vi "SVFA Convert FFT Spectrum to Custom Bandwidth Spectrum (1 Ch).vi"(0 "spectrum":cluster{"x0":dbl, "dx":dbl, "magnitude":dbl[]} {"magnitude" format="%.2f"; "dx" format="%.2f"; "x0" format="%.2f"}, 1 "frequency resolution profile in":cluster{"f center":dbl, "bandwidth":dbl}[](array[cluster])=[{"f center"=0.0, "bandwidth"=6.25}, {"f center"=1600.0, "bandwidth"=6.25}, {"f center"=1600.0, "bandwidth"=12.5}, {"f center"=3200.0, "bandwidth"=12.5}, {"f center"=3200.0, "bandwidth"=25.0}, {"f center"=6400.0, "bandwidth"=25.0}, {"f center"=6400.0, "bandwidth"=50.0}, {"f center"=12800.0, "bandwidth"=50.0}, {"f center"=12800.0, "bandwidth"=100.0}, {"f center"=20000.0, "bandwidth"=100.0}], 4 "spectrum info in":T1={"channel name"="", "description"="", "x-axis units"=0, "spectral info"={"spectrum type"=enum."Power [Magnitude^2]", "linear/dB"=enum."linear", "window"=0, "window size"=0, "FFT size"=0}, "engineering units"=0, "custom label"="", "dB reference [EU]"=0.0, "peak units"=enum."rms", "weighting filter"=0, "spectral density?"=FALSE, "unit label"="", "spectrum skewed?"=FALSE, "complimentary spectrum units"=enum."none"} {"x-axis units" items=["Time (s)"=0, "Frequency-CB (Hz)"=1, "Frequency-CPB (Hz)"=1248, "Frequency-Arbitrary (Hz)"=2357, "Quefrency (s)"=2, "Revolutions (rev)"=3, "Order"=4, "Speed (RPM)"=11, "Speed (rad/s)"=21, "Index"=65535]; "weighting filter" items=["Linear", "A-weighting", "B-weighting", "C-weighting", "ITU-R 468-4", "Dolby", "CCITT", "C-message", "Wb", "Wc", "Wd", "We", "Wf", "Wh", "Wj", "Wk", "Wm", "AES17 20 kHz lowpass", "AES17 40 kHz lowpass", "AES17 20 kHz highpass", "AES17 40 kHz highpass"]; "dB reference [EU]" format="%.2f"; "engineering units" items=["custom..."=0, "V"=1, "A"=21, "C"=30, "pC"=31, "s"=32, "-"=29, "Pa"=2, "N"=20, "g"=3, "m/s^2"=4, "m/s"=5, "m"=6, "mm/s"=12, "mm"=13, "micron/s"=14, "micron"=15, "in/s^2"=7, "in/s"=8, "in"=9, "mil/s"=10, "mil"=11, "rad/s^2"=16, "rad/s"=17, "rad"=18, "deg/s^2"=26, "deg/s"=27, "deg"=28, "RPM"=22, "cycle/s^2"=23, "Hz"=24, "cycle"=25, "strain"=19]; "spectral info"."window" items=["None "=0, "Hanning"=1, "Hamming"=2, "Blackman-Harris"=3, "Exact Blackman"=4, "Blackman"=5, "Flat Top"=6, "4 Term B-Harris "=7, "7 Term B-Harris"=8, "Low Sidelobe"=9, "Force - Exponential"=10, "Gaussian"=62]}, 5 "error in (no error)":errorcluster) -> (14 "spectrum":cluster{"frequencies [Hz]":dbl[], "power":dbl[]} {"power" format="%.2f"; "frequencies [Hz]" format="%.2f"}, 15 "unit label":string, 16 "total band power":dbl=nan format="%.2f", 18 "spectrum info out":T1={"channel name"="", "description"="", "x-axis units"=0, "spectral info"={"spectrum type"=enum."Power [Magnitude^2]", "linear/dB"=enum."linear", "window"=0, "window size"=0, "FFT size"=0}, "engineering units"=0, "custom label"="", "dB reference [EU]"=0.0, "peak units"=enum."rms", "weighting filter"=0, "spectral density?"=FALSE, "unit label"="", "spectrum skewed?"=FALSE, "complimentary spectrum units"=enum."none"} {"x-axis units" items=["Time (s)"=0, "Frequency-CB (Hz)"=1, "Frequency-CPB (Hz)"=1248, "Frequency-Arbitrary (Hz)"=2357, "Quefrency (s)"=2, "Revolutions (rev)"=3, "Order"=4, "Speed (RPM)"=11, "Speed (rad/s)"=21, "Index"=65535]; "weighting filter" items=["Linear", "A-weighting", "B-weighting", "C-weighting", "ITU-R 468-4", "Dolby", "CCITT", "C-message", "Wb", "Wc", "Wd", "We", "Wf", "Wh", "Wj", "Wk", "Wm", "AES17 20 kHz lowpass", "AES17 40 kHz lowpass", "AES17 20 kHz highpass", "AES17 40 kHz highpass"]; "dB reference [EU]" format="%.2f"; "engineering units" items=["custom..."=0, "V"=1, "A"=21, "C"=30, "pC"=31, "s"=32, "-"=29, "Pa"=2, "N"=20, "g"=3, "m/s^2"=4, "m/s"=5, "m"=6, "mm/s"=12, "mm"=13, "micron/s"=14, "micron"=15, "in/s^2"=7, "in/s"=8, "in"=9, "mil/s"=10, "mil"=11, "rad/s^2"=16, "rad/s"=17, "rad"=18, "deg/s^2"=26, "deg/s"=27, "deg"=28, "RPM"=22, "cycle/s^2"=23, "Hz"=24, "cycle"=25, "strain"=19]; "spectral info"."window" items=["None "=0, "Hanning"=1, "Hamming"=2, "Blackman-Harris"=3, "Exact Blackman"=4, "Blackman"=5, "Flat Top"=6, "4 Term B-Harris "=7, "7 Term B-Harris"=8, "Low Sidelobe"=9, "Force - Exponential"=10, "Gaussian"=62]}, 19 "error out":errorcluster)   [LabVIEW 2017]
doc: "Computes the aggregate power in the <B>range</B>. The SVL Power in Band VI operates on Power, PSD, COP, and FFT [Mag] spectra. You can use this polymorphic VI to analyze a single spectrum or N spectra. The data type you wire to the <B>spectrum</B> input determines the polymorphic instance to use."
uses:
  <vilib>/addons/_NISVFA/_Shared subVIs/Controls/svc_Spectrum Info.ctl
  <vilib>/addons/_NISVFA/_Shared subVIs/Controls/svc_X-Axis Units.ctl
  <vilib>/addons/_NISVFA/_Shared subVIs/Controls/svc_Spectrum Type.ctl
  <vilib>/addons/_NISVFA/_Shared subVIs/Controls/svc_Engineering Units Text Ring.ctl
  <vilib>/addons/_NISVFA/_Shared subVIs/Controls/svc_Weighting Filter Text Ring.ctl
  <vilib>/addons/_NISVFA/_Shared subVIs/Controls/svc_Complimentary Spectrum Units.ctl
  <vilib>/addons/_NISVFA/_Spectrum Processing/SVFA Unit Conversion (1 Ch).vi
  <vilib>/addons/_NISVFA/_Spectrum Processing/subVIs/svfa_Conversion Utility (spectrum info).vi
  <vilib>/addons/_NISVFA/_Spectrum Processing/subVIs/svfa_Peak to RMS to Peak2Peak.vi
  <vilib>/addons/_NISVFA/_Spectrum Processing/subVIs/svfa_Mag to Mag2.vi
  <vilib>/addons/_NISVFA/_Spectrum Processing/subVIs/svfa_Linear to dB.vi
  <vilib>/addons/_NISVFA/_Spectrum Processing/subVIs/svfa_dBrefA to dBrefB.vi
  <vilib>/addons/_NISVFA/_Spectrum Processing/subVIs/svfa_Spectrum to Spectral Density.vi
  <vilib>/addons/_NISVFA/_Shared subVIs/Common/svc_Get Weighting Enum and Labels.vi
  <vilib>/addons/_NISVFA/_Shared subVIs/Common/svc_Unit Label Lexical Class.vi
  <vilib>/addons/_NISVFA/_Shared subVIs/Common/svc_Engineering Units to Unit Label.vi
  <vilib>/addons/_NISVFA/_Shared subVIs/Common/svc_Format Value (DBL).vi
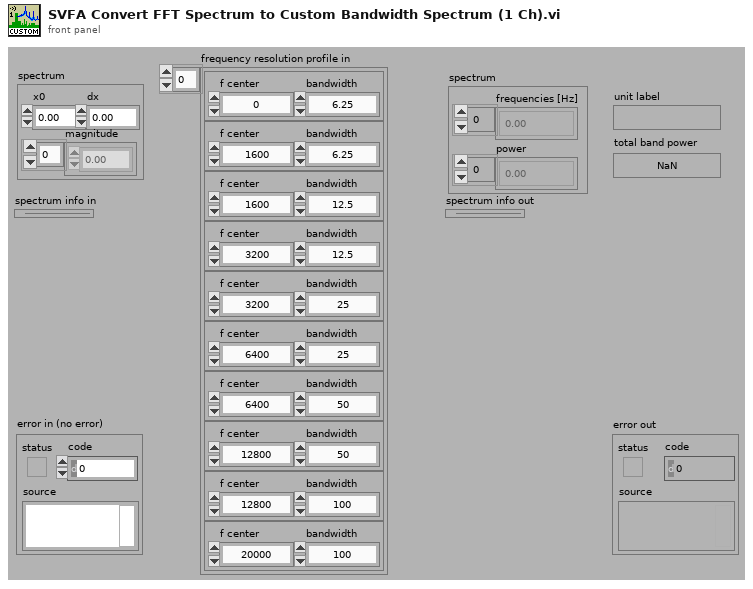
[diagram p1: front panel]
types:
  T1 = typedef "svc_Spectrum Info.ctl" = cluster{"channel name":string, "description":string, "x-axis units":T2, "spectral info":cluster{"spectrum type":T3, "linear/dB":enum16{"linear", "dB"}, "window":u16, "window size":i32, "FFT size":i32}, "engineering units":T4, "custom label":string, "dB reference [EU]":dbl, "peak units":enum16{"rms", "peak", "peak-peak"}, "weighting filter":T5, "spectral density?":bool, "unit label":string, "spectrum skewed?":bool, "complimentary spectrum units":T6}
  T2 = typedef "svc_X-Axis Units.ctl" = u16
  T3 = typedef "svc_Spectrum Type.ctl" = enum16{"FFT Spectrum [complex]", "Amplitude [Magnitude]", "Power [Magnitude^2]", "Cross Spectrum [complex]", "Frequency Response [Complex]"}
  T4 = typedef "svc_Engineering Units Text Ring.ctl" = u16
  T5 = typedef "svc_Weighting Filter Text Ring.ctl" = u16
  T6 = typedef "svc_Complimentary Spectrum Units.ctl" = enum16{"none", "radians", "degrees", "cycles", "imaginary"}
  T7 = cluster{"linear/dB":enum16{"no change", "linear", "dB"}, "dB reference (0: no change)":dbl, "power/magnitude":enum16{"no change", "power", "magnitude"}, "view":enum16{"no change", "rms", "peak", "peak-peak"}}
  T8 = enum16{"no change", "spectrum", "spectral density"}
  T9 = cluster{"f low":dbl, "f high":dbl, "f center":dbl, "bandwidth":dbl}[]
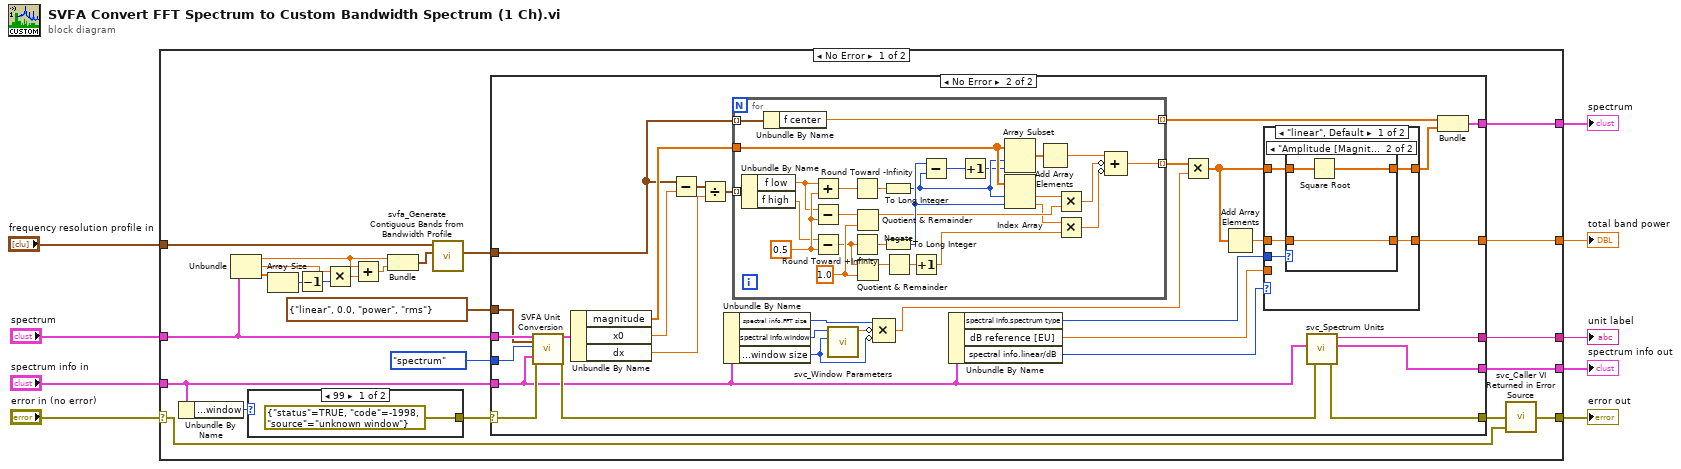
[diagram p0: block diagram]
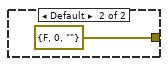
[diagram p2: hidden frame]
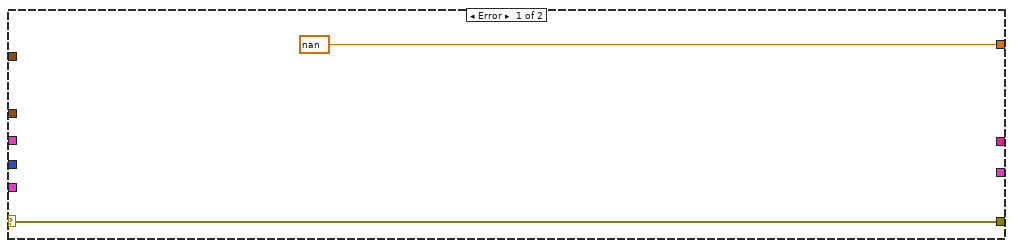
[diagram p3: hidden frame]
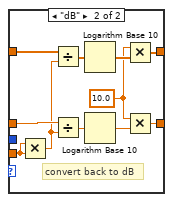
[diagram p5: hidden frame]
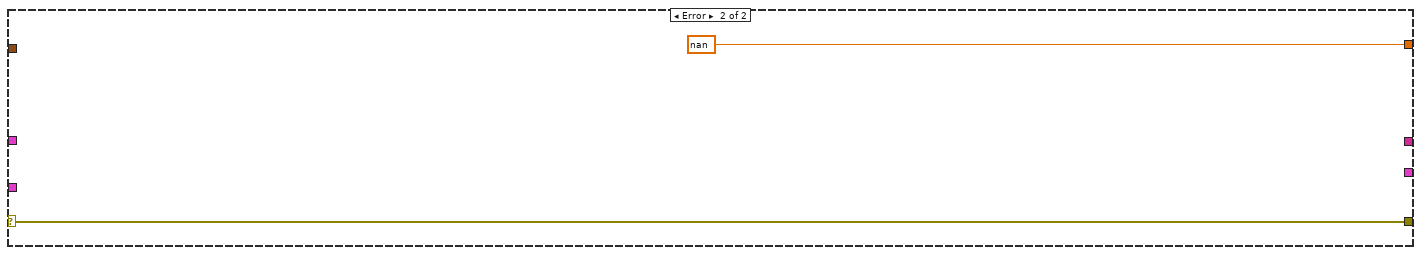
[diagram p6: hidden frame]
diagram:
  n1 = case shown="No Error" "error in (no error)" {
    selector: "error in (no error)" -> [w24 w118]
    tunnel: "spectrum" -> [w20 _]
    tunnel: [w31 nan ("power in band")] -> w8
    tunnel: [w32 w118] -> w7
    tunnel: "spectrum info in" -> [w21 _]
    tunnel: [w18 _] -> w5
    tunnel: [w19 _] -> w3
    tunnel: [w17 _] -> w2
    tunnel: "frequency resolution profile in" -> [w14 _]
    frame No Error {
      n2 = Unbundle By Name(w21) -> ("spectral info.window"=w22:u16)
      n3 = Unbundle(w20) -> ("x0"=w13:dbl, "dx"=w25:dbl, "magnitude"=w29:dbl[])
      n4 = case shown="99" w22 {
        tunnel: [errorcluster {"status"=TRUE, "code"=-1998, "source"="unknown window"} ("error out") errorcluster {"status"=FALSE, "code"=0, "source"=""} ("error out")] -> w23
        frame 99 {
        }
        frame Default {
        }
      }
      n5 = Array Size(array=w29) -> (size(s)=w27:i32)
      n6 = Decrement(x=w27) -> (x-1=w26:i32)
      n7 = Multiply(x=w25, y=w26) -> (x*y=w28:dbl)
      n8 = Add(x=w13, y=w28) -> (x+y=w12:dbl)
      n9 = Bundle("x0"=w13, w12) -> (w11:cluster{"x0":dbl, dbl})  [unwired: 1 in]
      n10 = call <vilib>:"svfa_Generate Contiguous Bands from Bandwidth Profile.vi"("frequency range [Hz]"=w11, "frequency resolution profile in"=w14) -> ("band specifications [Hz]"=w10:T9)  [unwired: 8 in, 1 out]
      n11 = case shown="No Error" w23 {
        selector: w23 -> [w36 w59]
        tunnel: w20 -> [_ w65]
        tunnel: w21 -> [_ w37]
        tunnel: [nan w60] -> w31
        tunnel: [w36 w40] -> w30
        tunnel: [_ w58] -> w19
        tunnel: [_ w41] -> w18
        tunnel: [_ w42] -> w17
        tunnel: T7 {"linear/dB"=enum."linear", "dB reference (0: no change)"=0.0, "power/magnitude"=enum."power", "view"=enum."rms"} ("desired scaling") -> [_ w57]
        tunnel: T8."spectrum" ("spectral density desired") -> [_ w56]
        tunnel: w10 -> [_ w39]
        frame Error {
        }
        frame No Error {
          n12 = call-poly <vilib>:"SVFA Unit Conversion.vi"("spectrum"=w65, "desired scaling"=w57, "spectral density desired"=w56, "spectrum info in"=w37, "error in (no error)"=w59) -> ("converted spectrum"=w67:cluster{"x0":dbl, "dx":dbl, "magnitude":dbl[]}, "error out"=w43:errorcluster)  [unwired: 11 in, 2 out]
          n13 = Unbundle By Name(w67) -> ("magnitude"=w46:dbl[], "x0"=w64:dbl, "dx"=w63:dbl)
          n14 = Subtract(x=w39, y=w64) -> (x-y=w66:T9)
          n15 = Divide(x=w66, y=w63) -> (x/y=w47:T9)
          n16 = Unbundle By Name(w37) -> ("spectral info.FFT size"=w52:i32, "spectral info.window"=w53:u16, "spectral info.window size"=w50:i32)
          n17 = for {
            tunnel: w47 -> [w95] mode=indexing
            tunnel: w46 -> [w94]
            tunnel: [w93] -> w45 mode=indexing
            tunnel: w39 -> [w76] mode=indexing
            tunnel: [w75] -> w38 mode=indexing
            w84 = 0.5 ("x")
            w88 = 1.0 ("y")
            n18 = Unbundle By Name(w95) -> ("f low"=w77:dbl, "f high"=w78:dbl)
            n19 = Unbundle By Name(w76) -> ("f center"=w75:dbl)
            n20 = Add(x=w77, y=w84) -> (x+y=w91:dbl)
            n21 = Subtract(x=w77, y=w84) -> (x-y=w85:dbl)
            n22 = Subtract(x=w78, y=w84) -> (x-y=w81:dbl)
            n23 = Round Toward -Infinity(1:w91) -> (0:w90:dbl)
            n24 = Round Toward +Infinity(x=w81) -> (ceil(x): smallest int >= x=w92:dbl)
            n25 = Quotient & Remainder(x=w85, y=w88) -> (x-y*floor(x/y)=w80:dbl)  [unwired: 1 out]
            n26 = Quotient & Remainder(x=w81, y=w88) -> (x-y*floor(x/y)=w83:dbl)  [unwired: 1 out]
            n27 = To Long Integer(number=w90) -> (32bit integer=w87:i32)
            n28 = To Long Integer(number=w92) -> (32bit integer=w89:i32)
            n29 = Negate(x=w83) -> (-x=w82:dbl)
            n30 = Increment(x=w82) -> (x+1=w79:dbl)
            n31 = Subtract(x=w89, y=w87) -> (x-y=w86:i32)
            n32 = Increment(x=w86) -> (x+1=w70:i32)
            n33 = Array Subset(array=w94, index=w87, length=w70) -> (w71:dbl[])
            n34 = Index Array(array=w94, index #1=w87, index #2=w89) -> (element #1=w69:dbl, element #2=w68:dbl)
            n35 = Add Array Elements(numeric array=w71) -> (sum=w74:dbl)
            n36 = Multiply(x=w69, y=w80) -> (x*y=w73:dbl)
            n37 = Multiply(x=w68, y=w79) -> (x*y=w72:dbl)
            n38 = Compound Arithmetic op=ADD(w74, invert w73, invert w72) -> (w93:dbl)
          }
          n39 = call <vilib>:"svc_Window Parameters.vi"("window size"=w50, "window"=w53) -> ("ENBW"=w51:dbl)  [unwired: 6 in, 3 out]
          n40 = Compound Arithmetic op=MULTIPLY(w52, invert w51, invert w50) -> (w49:dbl)
          n41 = Unbundle By Name(w37) -> ("spectral info.spectrum type"=w44:T3, "dB reference [EU]"=w55:dbl, "spectral info.linear/dB"=w54:enum16{"linear", "dB"})
          n42 = Multiply(x=w45, y=w49) -> (x*y=w48:dbl[])
          n43 = Add Array Elements(numeric array=w48) -> (sum=w61:dbl)
          n44 = case shown="\"linear\", Default" w54 {
            tunnel: [w97 w116] -> w62
            tunnel: w48 -> [w98 w114]
            tunnel: w55 -> [_ w112]
            tunnel: w61 -> [w99 w109]
            tunnel: [w96 w107] -> w60
            tunnel: w44 -> [w100 _]
            frame "linear", Default {
              n45 = case shown="\"Amplitude [Magnitude]\"" w100 {
                tunnel: w99 -> [w101 w104]
                tunnel: w98 -> [w102 w105]
                tunnel: [w102 w103] -> w97
                tunnel: [w101 w104] -> w96
                frame "Power [Magnitude^2]", Default {
                }
                frame "Amplitude [Magnitude]" {
                  n46 = Square Root(x=w105) -> (sqrt(x)=w103:dbl[])
                }
              }
            }
            frame "dB" {
              w106 = 10.0 ("Numeric")
              # "convert back to dB"
              n47 = Multiply(x=w112, y=w112) -> (x*y=w108:dbl)
              n48 = Divide(x=w114, y=w108) -> (x/y=w113:dbl[])
              n49 = Divide(x=w109, y=w108) -> (x/y=w111:dbl)
              n50 = Logarithm Base 10(1:w113) -> (0:w115:dbl[])
              n51 = Logarithm Base 10(1:w111) -> (0:w110:dbl)
              n52 = Multiply(x=w106, y=w115) -> (x*y=w116:dbl[])
              n53 = Multiply(x=w106, y=w110) -> (x*y=w107:dbl)
            }
          }
          n54 = call <vilib>:"svc_Spectrum Units.vi"("error in (no error)"=w43, "spectrum info in"=w37) -> ("error out"=w40:errorcluster, "spectrum info out"=w42:T1, "unit label"=w41:string)  [unwired: 2 in, 1 out]
          n55 = Bundle(w38, w62) -> (w58:cluster{dbl[], dbl[]})  [unwired: 1 in]
        }
      }
      n56 = call <vilib>:"svc_Caller VI Returned in Error Source.vi"("warning input to caller"=w24, "error in (no error)"=w30) -> ("error out"=w32:errorcluster)  [unwired: 3 in]
    }
    frame Error {
    }
  }
  "error out" <- w7
  "total band power" <- w8
  "unit label" <- w5
  "spectrum" <- w3
  "spectrum info out" <- w2
